vi "CheckCollision.vi"(0 "object in":refnum<class "Battleship.lvclass">, 2 "Battleship":refnum<class "Battleship.lvclass">, 5 "error in (no error)":errorcluster) -> (14 "object out":refnum<class "Battleship.lvclass">, 16 "Collision?":bool, 19 "error out":errorcluster)   [LabVIEW 2015, in "Battleship.lvclass"]
doc: "Returns true if the battleships positions collide with each other. Ships need to be at least 1 square in each direction away from each other."
uses:
  Battleship.lvclass
  TypDefs/Coordinates.ctl
  Battleship.lvclass/Battleship.ctl
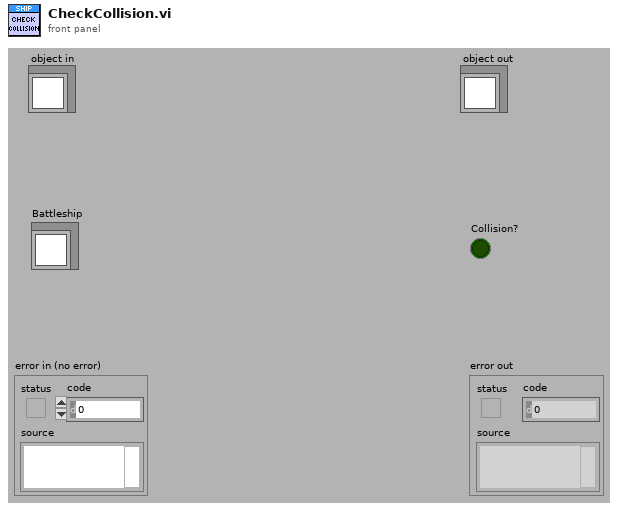
[diagram p1: front panel]
types:
  T1 = typedef "Coordinates.ctl" = cluster{"X":i32, "Y":i32}
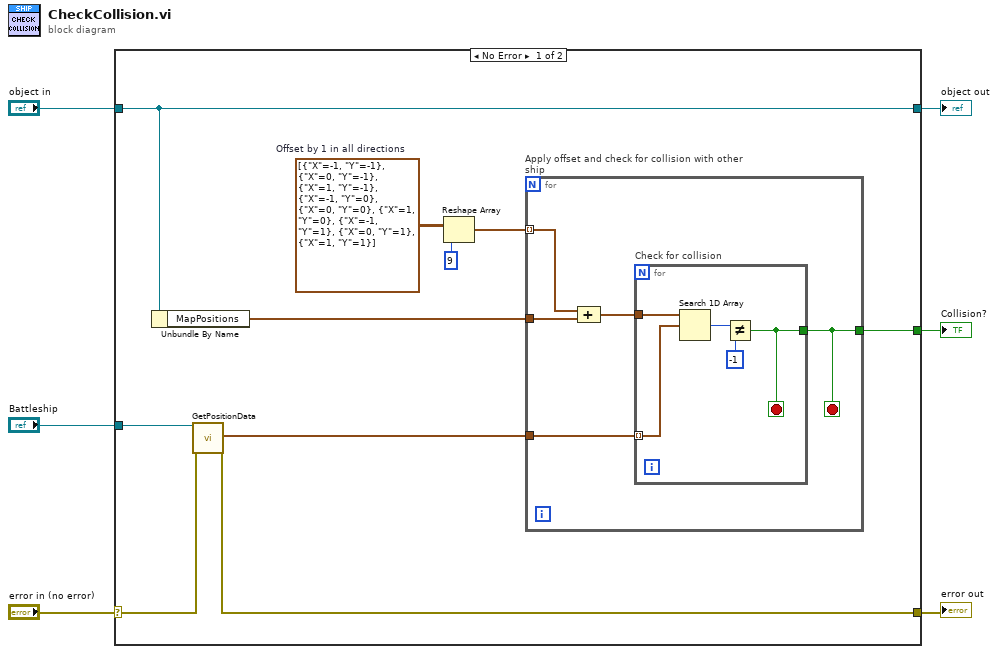
[diagram p0: block diagram]
diagram:
  n1 = case shown="No Error" "error in (no error)" {
    selector: "error in (no error)" -> [w14 w28]
    tunnel: [w13 w28] -> w5
    tunnel: [w16 w27] -> w3
    tunnel: "object in" -> [w16 w27]
    tunnel: "Battleship" -> [w15 _]
    tunnel: [w10 _] -> w1
    frame No Error {
      w9 = T1[][] [[{"X"=-1, "Y"=-1}, {"X"=0, "Y"=-1}, {"X"=1, "Y"=-1}], [{"X"=-1, "Y"=0}, {"X"=0, "Y"=0}, {"X"=1, "Y"=0}], [{"X"=-1, "Y"=1}, {"X"=0, "Y"=1}, {"X"=1, "Y"=1}]]  # Offset by 1 in all directions
      n2 = Unbundle By Name(w16) -> ("MapPositions"=w12:T1[])
      n3 = call-dynamic "GetPositionData.vi"("object in"=w15, "error in (no error)"=w14) -> ("MapPositions"=w11:T1[], "error out"=w13:errorcluster)  [unwired: 13 in, 3 out]
      n4 = Reshape Array(w9, 9 ("dimension size")) -> (w7:T1[])
      n5 = for "Apply offset and check for collision with other ship" {
        tunnel: w12 -> [w19]
        tunnel: w11 -> [w21]
        tunnel: [w20] -> w10
        tunnel: w7 -> [w17] mode=indexing
        stop <- w20 stop-if-true
        n6 = Compound Arithmetic op=unknown(w17, w19) -> (w18:T1[])
        n7 = for "Check for collision" {
          tunnel: w18 -> [w26]
          tunnel: w21 -> [w25] mode=indexing
          tunnel: [w22] -> w20
          stop <- w22 stop-if-true
          n8 = Search 1D Array(1D array=w26, element=w25) -> (index of element=w24:i32)  [unwired: 1 in]
          n9 = Not Equal?(x=w24, y=-1) -> (x != y?=w22:bool)
        }
      }
    }
    frame Error {
    }
  }
  "error out" <- w5
  "object out" <- w3
  "Collision?" <- w1
